vi "PLC.Global.vi"() -> ()   [LabVIEW 2016]
uses:
  PLC.Data.Status.ctl
  PLC.State.ctl
  PLC.Data.Sets.ctl
panel:
  in  "PLC3.Sets":T1={"Enable"=TRUE, "IP"="192.168.1.20", "Rack"=0, "Slot"=2, "LifeBitTimer_s"=15.0, "DataBlockAddr_PCStatus"=401, "DataBlockAddr_PLCStatus"=4, "DataBlockAddr_PLCNewData"=[], "DataBlockSize_PLCNewData"=[], "DataBlockAddr_PLCChangeOver"=[], "DataBlockSize_PLCChangeOver"=[], "DataBlockAddr_PCChangeOver"=[], "DataBlockAddr_PLCCheckStatus"=[], "DataBlockSize_PLCCheckStatus"=[], "DataBlockAddr_PCCheckStatus"=[], "System"=""}
  out "PLC3.Status":T2
  in  "PLC2.Sets":T1={"Enable"=TRUE, "IP"="192.168.1.20", "Rack"=0, "Slot"=2, "LifeBitTimer_s"=15.0, "DataBlockAddr_PCStatus"=401, "DataBlockAddr_PLCStatus"=4, "DataBlockAddr_PLCNewData"=[], "DataBlockSize_PLCNewData"=[], "DataBlockAddr_PLCChangeOver"=[], "DataBlockSize_PLCChangeOver"=[], "DataBlockAddr_PCChangeOver"=[], "DataBlockAddr_PLCCheckStatus"=[], "DataBlockSize_PLCCheckStatus"=[], "DataBlockAddr_PCCheckStatus"=[], "System"=""}
  out "PLC2.Status":T2
  in  "PLC1.Sets":T1={"Enable"=TRUE, "IP"="192.168.1.20", "Rack"=0, "Slot"=2, "LifeBitTimer_s"=15.0, "DataBlockAddr_PCStatus"=401, "DataBlockAddr_PLCStatus"=4, "DataBlockAddr_PLCNewData"=[], "DataBlockSize_PLCNewData"=[], "DataBlockAddr_PLCChangeOver"=[], "DataBlockSize_PLCChangeOver"=[], "DataBlockAddr_PCChangeOver"=[], "DataBlockAddr_PLCCheckStatus"=[], "DataBlockSize_PLCCheckStatus"=[], "DataBlockAddr_PCCheckStatus"=[], "System"=""}
  out "PLC1.Status":T2
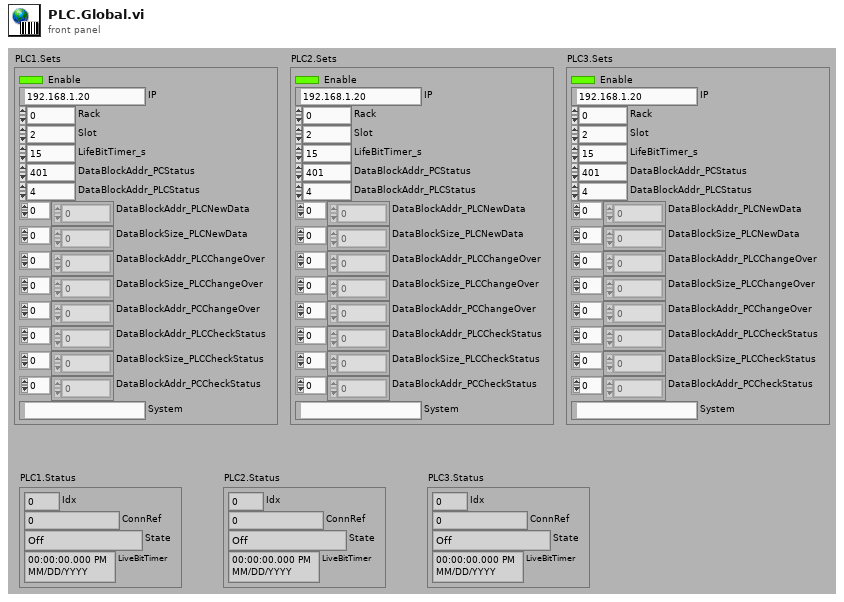
[diagram p1: front panel]
types:
  T1 = typedef "PLC.Data.Sets.ctl" = cluster{"Enable":bool, "IP":string, "Rack":i32, "Slot":i32, "LifeBitTimer_s":dbl, "DataBlockAddr_PCStatus":i32, "DataBlockAddr_PLCStatus":i32, "DataBlockAddr_PLCNewData":i32[], "DataBlockSize_PLCNewData":i32[], "DataBlockAddr_PLCChangeOver":i32[], "DataBlockSize_PLCChangeOver":i32[], "DataBlockAddr_PCChangeOver":i32[], "DataBlockAddr_PLCCheckStatus":i32[], "DataBlockSize_PLCCheckStatus":i32[], "DataBlockAddr_PCCheckStatus":i32[], "System":string}
  T2 = typedef "PLC.Data.Status.ctl" = cluster{"Idx":i32, "ConnRef":u64, "State":T3, "LiveBitTimer":timestamp}
  T3 = typedef "PLC.State.ctl" = enum32{"Off", "Error", "Idle", "Run"}
diagram:
